vi "file an issue dialog.vi"() -> ()   [LabVIEW 2016, in "FPGA Resource Manager System Defintion.lvlib"]
uses:
  FPGA Resource Manager System Defintion.lvlib
  <vilib>/NI/JSON Support for LabVIEW/JSON Value/New JSON Value/New JSON ({String[]}).vi
  <vilib>/httpClient/POSTBuffer.vi
  <vilib>/NI/JSON Support for LabVIEW/JSON Value/JSON Value.lvclass
  <vilib>/httpClient/LabVIEWHTTPClient.lvlib
panel:
  in  "your name":string
  in  "url":string="https://api.github.com/repos/LRUArchitecture/VeriStand-FPGA-Resource-Manager/issues"
  out "body 2":string
  out "String":string
  in  "body":string
  in  "title (Required)":string
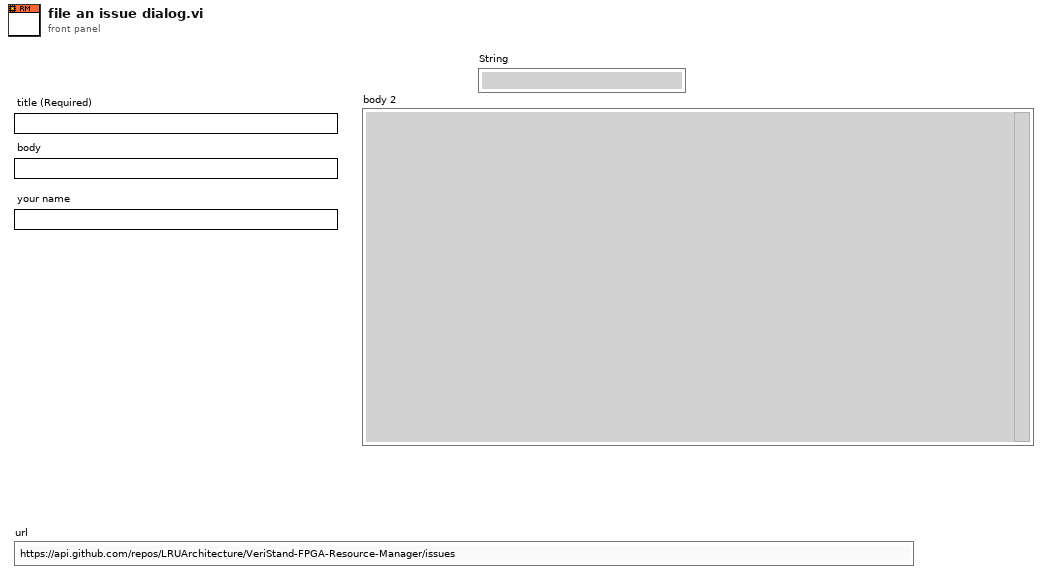
[diagram p1: front panel]
types:
  T1 = typedef "LabVIEWHTTPClient.lvlib/ClientHandle.ctl" = refnum<k1>
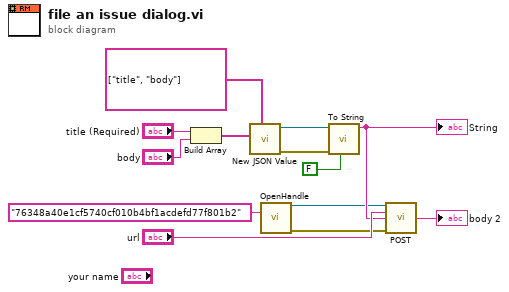
[diagram p0: block diagram]
diagram:
  n1 = Build Array("title (Required)", "body") -> (w10:string[])
  n2 = call-poly <vilib>:"New JSON Value.vi"("keys"=string[] ["title", "body"] ("key"), "values"=w10) -> ("error out"=w9:errorcluster, "JSON Value out"=w8:refnum<class "JSON Value.lvclass">)  [unwired: 8 in]
  n3 = call <vilib>:"OpenHandle.vi"("username"="76348a40e1cf5740cf010b4bf1acdefd77f801b2") -> ("client handle out"=w3:T1, "error out"=w2:errorcluster)  [unwired: 13 in]
  n4 = call <vilib>:"To String.vi"("pretty print? (T)"=FALSE, "error in (no error)"=w9, "JSON Value in"=w8) -> ("String"=w5:string)  [unwired: 7 in, 1 out]
  "String" <- w5
  n5 = call-poly <vilib>:"POST.vi"("client handle"=w3, "url"="url", "buffer"=w5, "error in (no error)"=w2) -> ("body"=→"body 2":string)  [unwired: 8 in, 3 out]
